vi "FPGA Modular.vi"() -> ()   [LabVIEW 2014]
uses:
  SLSC FPGA Inputs.ctl
  <userlib>/_NI SPI IP/FPGA/Controllers/Public/Transfer Settings.ctl
  SLSC version.ctl
  SLSC FIFO name.ctl
  SLSC # of racks.ctl
  SLSC SPI Digital IO Lines.ctl
  <vilib>/rvi/Emulation/niFpgaGetClockAttributes.vi
  <vilib>/rvi/Emulation/niFpgaSctlEmulationGetInTimedLoop.vi
  <vilib>/rvi/Emulation/niFpgaEmulationReportErrorSimple.vi
  <vilib>/rvi/interface/RandomDataEmulation/niFpgaRandomDataHandleErrors.vi
  <vilib>/rvi/Emulation/niFpgaCriticalErrorInLSC.vi
  <vilib>/rvi/DataTransferAndStorage/Container/XNode/niFpgaContainer.xnode
  <vilib>/rvi/interface/RandomDataEmulation/nirviRandomDataFpgaReadWriteTemplate.vi
  SLSC FPGA Toolkit.lvlib
  <userlib>/_NI SPI IP/FPGA/Controllers/NI SPI IP FPGA.lvlib
panel:
  in  "slsc.# of Racks.4":T1
  in  "slsc.FIFO Name.SPI CMD FIFO":T2
  in  "slsc.version":T3
  in  "settings.SLSC":T4={"SPI PHY Settings"={"Divide Value"=20, "Transfer Length (bits)"=32, "CS Asserted Polarity"=FALSE, "Clock Polarity (CPOL)"=FALSE, "Clock Phase (CPHA)"=FALSE, "Lengthen MISO Setup"=FALSE, "Direction Change Bit"=0, "MOSI Starts as Output"=FALSE, "Tristatable MOSI"=FALSE}, "Sample Rate (S/s)"=10000} {"SPI PHY Settings"."Direction Change Bit" max=64 step=1; "SPI PHY Settings"."Transfer Length (bits)" min=1 max=64 step=1}
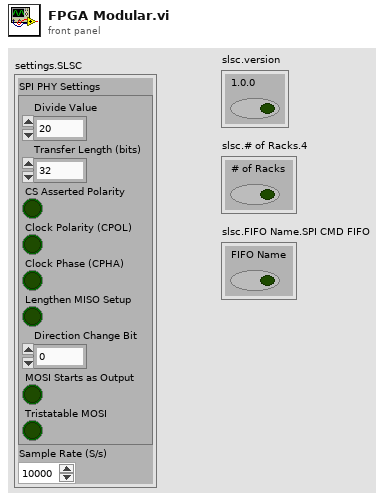
[diagram p1: front panel]
types:
  T1 = typedef "SLSC FPGA Toolkit.lvlib/SLSC # of racks.ctl" = cluster{"# of Racks":bool}
  T2 = typedef "SLSC FPGA Toolkit.lvlib/SLSC FIFO name.ctl" = cluster{"FIFO Name":bool}
  T3 = typedef "SLSC FPGA Toolkit.lvlib/SLSC version.ctl" = cluster{"1.0.0":bool}
  T4 = typedef "SLSC FPGA Toolkit.lvlib/SLSC FPGA Inputs.ctl" = cluster{"SPI PHY Settings":T5, "Sample Rate (S/s)":u32}
  T5 = typedef "NI SPI IP FPGA.lvlib/Transfer Settings.ctl" = cluster{"Divide Value":u8, "Transfer Length (bits)":u8, "CS Asserted Polarity":bool, "Clock Polarity (CPOL)":bool, "Clock Phase (CPHA)":bool, "Lengthen MISO Setup":bool, "Direction Change Bit":u8, "MOSI Starts as Output":bool, "Tristatable MOSI":bool}
  T6 = typedef "SLSC FPGA Toolkit.lvlib/SLSC SPI Digital IO Lines.ctl" = cluster{"SCLK":refnum<k21>, "MISO":refnum<k21>, "MOSI":refnum<k21>, "!Enable":refnum<k21>, "CS Bit 1":refnum<k21>, "CS Bit 2":refnum<k21>, "CS Bit 3":refnum<k21>, "CS Bit 4":refnum<k21>}
  T7 = typedef "SLSC configuration Shared.lvlib/CS Bits.ctl" = cluster{"CS Bit 1":refnum<k21>, "CS Bit 2":refnum<k21>, "CS Bit 3":refnum<k21>, "CS Bit 4":refnum<k21>}
  T8 = typedef "Internal Data (SPI API).ctl" = cluster{"DLU To SPI Engine Data FIFO":refnum<k21>, "SPI Engine to DLU Data FIFO":refnum<k21>, "Data to SPI Engine (Cache) Register":refnum<k21>, "SPI PHY Settings to SPI Engine (Cahche) Register":refnum<k21>}
  T9 = typedef "SPI Digital IO Lines.ctl" = cluster{"SCLK":refnum<k21>, "MISO":refnum<k21>, "MOSI":refnum<k21>, "CS 0":refnum<k21>, "CS 1":refnum<k21>, "CS 2":refnum<k21>, "CS 3":refnum<k21>, "CS 4":refnum<k21>, "CS 5":refnum<k21>}
  T10 = typedef "SLSC FPGA Toolkit.lvlib/SLSC SPI Command.ctl" = cluster{"Chip Select":u8, "CS Bit Value/Slot #":u8, "SPI PHY Settings":T5, "Data to DAC":u64}
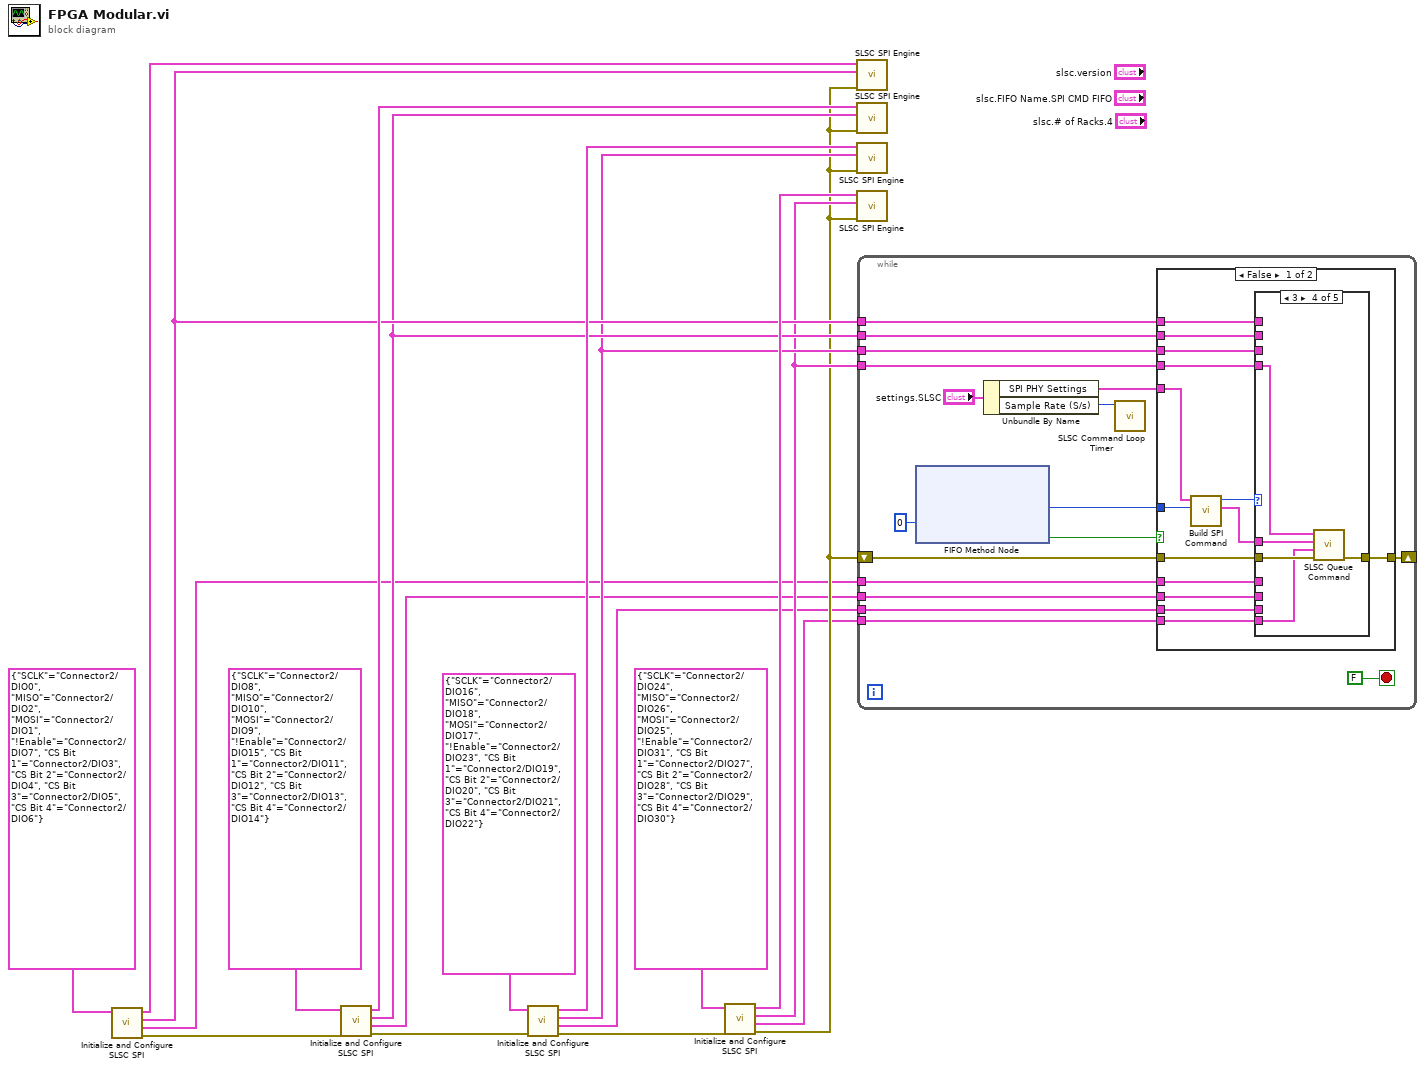
[diagram p0: block diagram]
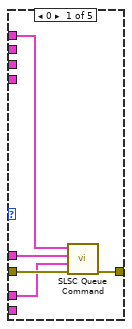
[diagram p2: hidden frame]
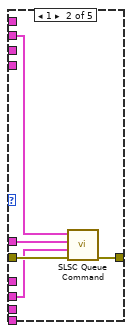
[diagram p3: hidden frame]
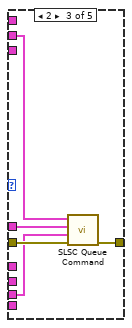
[diagram p4: hidden frame]
diagram:
  n1 = call "Initialize and Configure SLSC SPI.vi"("SLSC Chip Select DIO Lines"=T6 {"SCLK"="Connector2/DIO0", "MISO"="Connector2/DIO2", "MOSI"="Connector2/DIO1", "!Enable"="Connector2/DIO7", "CS Bit 1"="Connector2/DIO3", "CS Bit 2"="Connector2/DIO4", "CS Bit 3"="Connector2/DIO5", "CS Bit 4"="Connector2/DIO6"}) -> ("error out"=w17:errorcluster, "CS Bits"=w4:T7, "SPI API References"=w9:T8, "SPI DIO Lines"=w20:T9)  [unwired: 7 in]
  n2 = call "Initialize and Configure SLSC SPI.vi"("error in"=w17, "SLSC Chip Select DIO Lines"=T6 {"SCLK"="Connector2/DIO8", "MISO"="Connector2/DIO10", "MOSI"="Connector2/DIO9", "!Enable"="Connector2/DIO15", "CS Bit 1"="Connector2/DIO11", "CS Bit 2"="Connector2/DIO12", "CS Bit 3"="Connector2/DIO13", "CS Bit 4"="Connector2/DIO14"}) -> ("error out"=w15:errorcluster, "CS Bits"=w3:T7, "SPI API References"=w8:T8, "SPI DIO Lines"=w12:T9)  [unwired: 6 in]
  n3 = call "Initialize and Configure SLSC SPI.vi"("error in"=w15, "SLSC Chip Select DIO Lines"=T6 {"SCLK"="Connector2/DIO16", "MISO"="Connector2/DIO18", "MOSI"="Connector2/DIO17", "!Enable"="Connector2/DIO23", "CS Bit 1"="Connector2/DIO19", "CS Bit 2"="Connector2/DIO20", "CS Bit 3"="Connector2/DIO21", "CS Bit 4"="Connector2/DIO22"}) -> ("error out"=w14:errorcluster, "CS Bits"=w2:T7, "SPI API References"=w7:T8, "SPI DIO Lines"=w11:T9)  [unwired: 6 in]
  n4 = call "Initialize and Configure SLSC SPI.vi"("error in"=w14, "SLSC Chip Select DIO Lines"=T6 {"SCLK"="Connector2/DIO24", "MISO"="Connector2/DIO26", "MOSI"="Connector2/DIO25", "!Enable"="Connector2/DIO31", "CS Bit 1"="Connector2/DIO27", "CS Bit 2"="Connector2/DIO28", "CS Bit 3"="Connector2/DIO29", "CS Bit 4"="Connector2/DIO30"}) -> ("error out"=w5:errorcluster, "CS Bits"=w1:T7, "SPI API References"=w6:T8, "SPI DIO Lines"=w10:T9)  [unwired: 6 in]
  n5 = call "SLSC SPI Engine.vi"("error in (no error)"=w5, "SPI API References"=w9, "Chip Select DIO Lines"=w20) -> ()  [unwired: 9 in]
  n6 = call "SLSC SPI Engine.vi"("error in (no error)"=w5, "SPI API References"=w8, "Chip Select DIO Lines"=w12) -> ()  [unwired: 9 in]
  n7 = call "SLSC SPI Engine.vi"("error in (no error)"=w5, "SPI API References"=w7, "Chip Select DIO Lines"=w11) -> ()  [unwired: 9 in]
  n8 = call "SLSC SPI Engine.vi"("error in (no error)"=w5, "SPI API References"=w6, "Chip Select DIO Lines"=w10) -> ()  [unwired: 9 in]
  n9 = while {
    tunnel: w9 -> [w35]
    tunnel: w8 -> [w34]
    tunnel: w7 -> [w33]
    tunnel: w6 -> [w32]
    shift-right: [w30] -> _
    shift-left: w5 -> [w31]
    tunnel: w4 -> [w27]
    tunnel: w3 -> [w26]
    tunnel: w2 -> [w25]
    tunnel: w1 -> [w24]
    stop <- FALSE stop-if-true
    n10 = xnode ("FIFO Method Node")("Timeout"=0) -> ("Element"=w36:u64, "Timed Out?"=w28:bool)  [unwired: 1 in, 1 out]
    n11 = Unbundle By Name("settings.SLSC") -> ("SPI PHY Settings"=w22:T5, "Sample Rate (S/s)"=w21:u32)
    n12 = call "SLSC Command Loop Timer.vi"("inputs.Sample Rate (S/s)"=w21) -> ()  [unwired: 8 in, 3 out]
    n13 = case shown="False" w28 {
      tunnel: w36 -> [w51 _]
      tunnel: w22 -> [w50 _]
      tunnel: w35 -> [w47 _]
      tunnel: w34 -> [w46 _]
      tunnel: w33 -> [w45 _]
      tunnel: w32 -> [w44 _]
      tunnel: w31 -> [w43 w73]
      tunnel: [w42 w73] -> w30
      tunnel: w27 -> [w41 _]
      tunnel: w26 -> [w40 _]
      tunnel: w25 -> [w39 _]
      tunnel: w24 -> [w38 _]
      frame False {
        n14 = call "Build SPI Command.vi"("SPI CMD FIFO Element"=w51, "SPI PHY Settings"=w50) -> ("SLSC SPI Command"=w48:T10, "Rack #"=w49:u8)  [unwired: 8 in]
        n15 = case shown="3" w49 {
          tunnel: w48 -> [w56 w61 w66 w71 _]
          tunnel: w47 -> [w55 _ _ _ _]
          tunnel: w46 -> [_ w58 _ _ _]
          tunnel: w45 -> [_ _ w63 _ _]
          tunnel: w44 -> [_ _ _ w67 _]
          tunnel: w43 -> [w54 w60 w65 w70 w72]
          tunnel: [w53 w59 w64 w69 w72] -> w42
          tunnel: w41 -> [w52 _ _ _ _]
          tunnel: w40 -> [_ w57 _ _ _]
          tunnel: w39 -> [_ _ w62 _ _]
          tunnel: w38 -> [_ _ _ w68 _]
          frame 0 {
            n16 = call "SLSC Queue Command.vi"("error in"=w54, "CS Bits"=w52, "SLSC SPI Command"=w56, "SPI API References"=w55) -> ("error out"=w53:errorcluster)  [unwired: 5 in, 2 out]
          }
          frame 1 {
            n17 = call "SLSC Queue Command.vi"("error in"=w60, "CS Bits"=w57, "SLSC SPI Command"=w61, "SPI API References"=w58) -> ("error out"=w59:errorcluster)  [unwired: 5 in, 2 out]
          }
          frame 2 {
            n18 = call "SLSC Queue Command.vi"("error in"=w65, "CS Bits"=w62, "SLSC SPI Command"=w66, "SPI API References"=w63) -> ("error out"=w64:errorcluster)  [unwired: 5 in, 2 out]
          }
          frame 3 {
            n19 = call "SLSC Queue Command.vi"("error in"=w70, "CS Bits"=w68, "SLSC SPI Command"=w71, "SPI API References"=w67) -> ("error out"=w69:errorcluster)  [unwired: 5 in, 2 out]
          }
          frame Default {
          }
        }
      }
      frame True {
      }
    }
  }
